vi "_testStepCfgEditor.vi"() -> ()   [LabVIEW 2010]
panel:
  out "View row details":string[](array[string])
  in  "stop":bool
  in  "Library function":string(tree)="sigDirMulStatInSet"
  in  "Test Step CFG EDIT":string[][](table)
  out "error out":errorcluster
  in  "error in":errorcluster
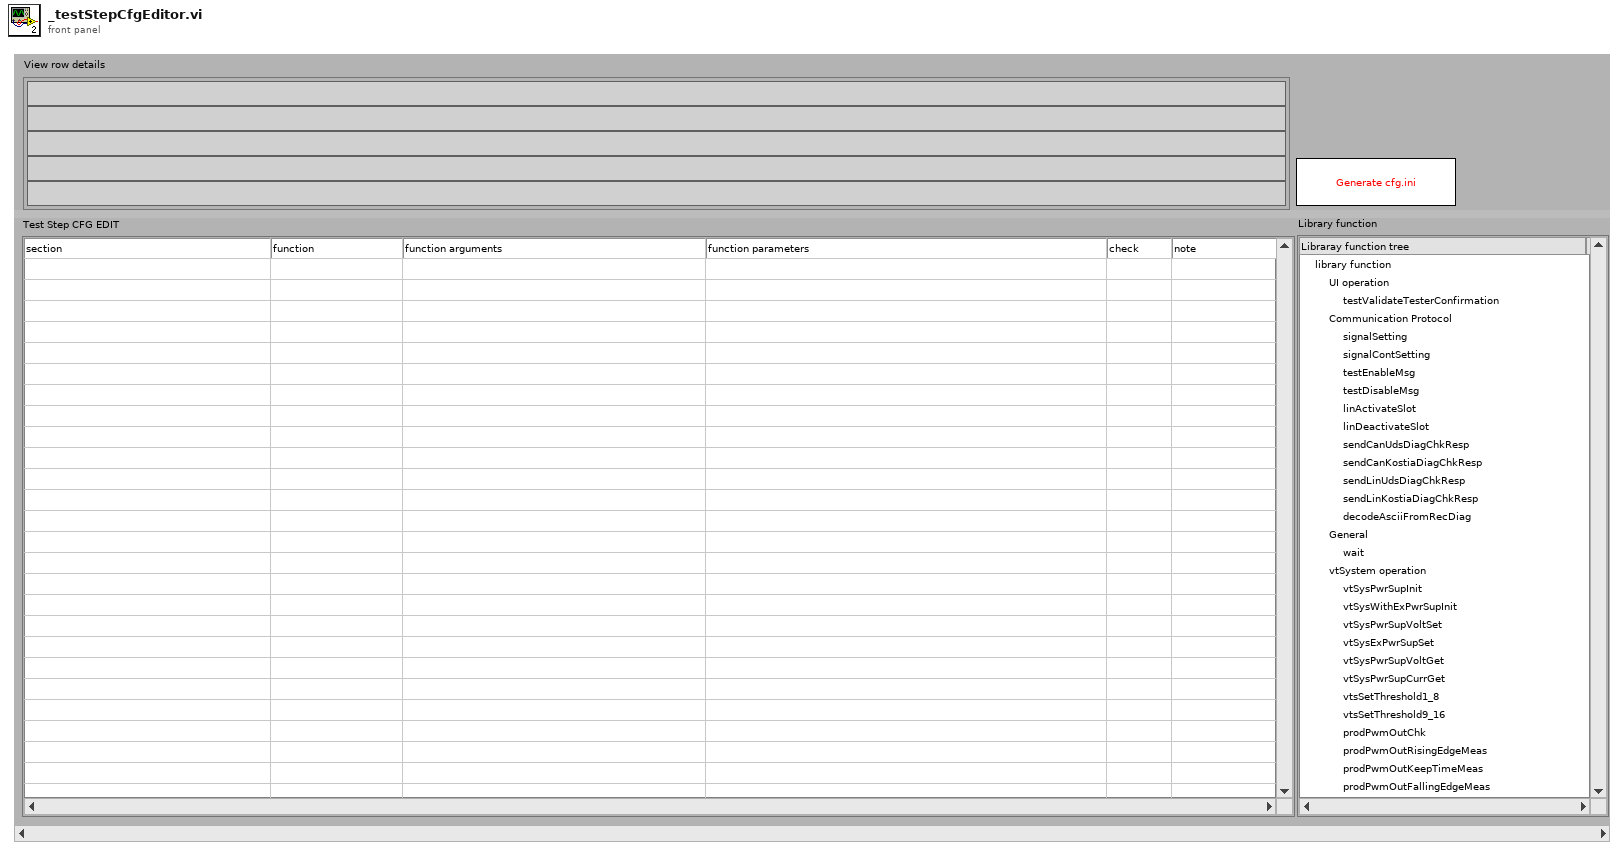
[diagram p1: front panel]
types:
  T1 = typedef "LVRowAndColumnTypeDef.ctl" = cluster{"Row":i32, "Column":i32}
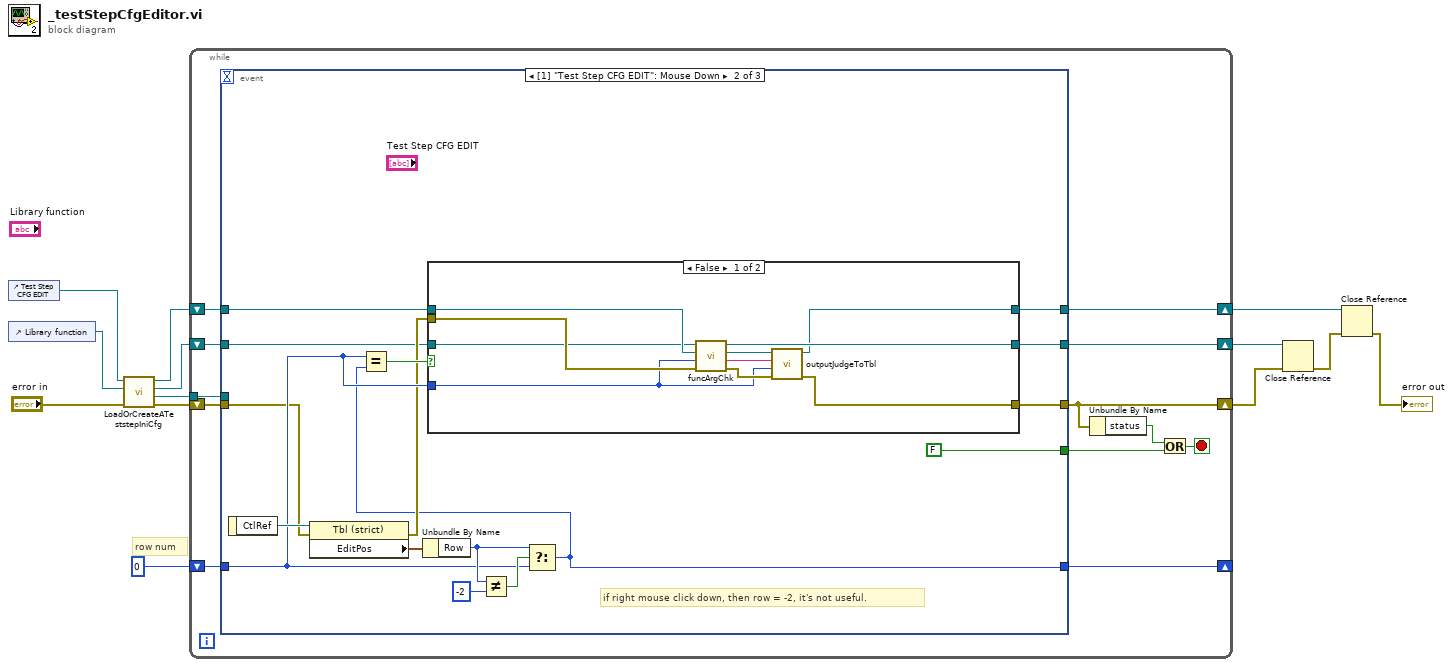
[diagram p0: block diagram]
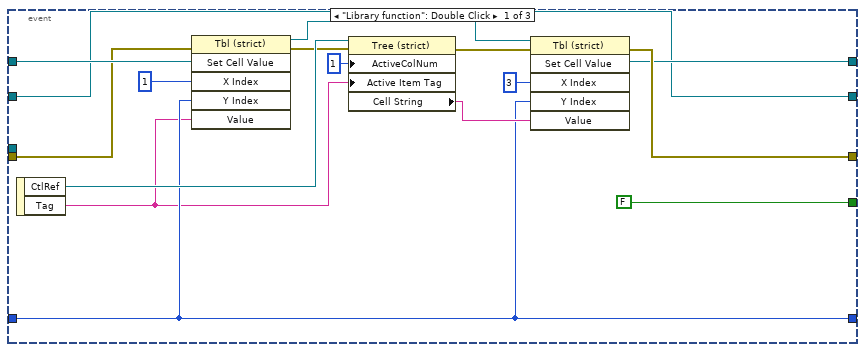
[diagram p2: hidden frame]
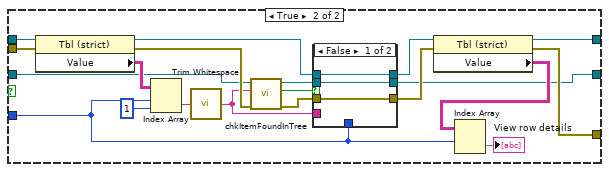
[diagram p3: hidden frame]
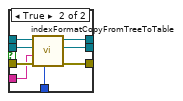
[diagram p4: hidden frame]
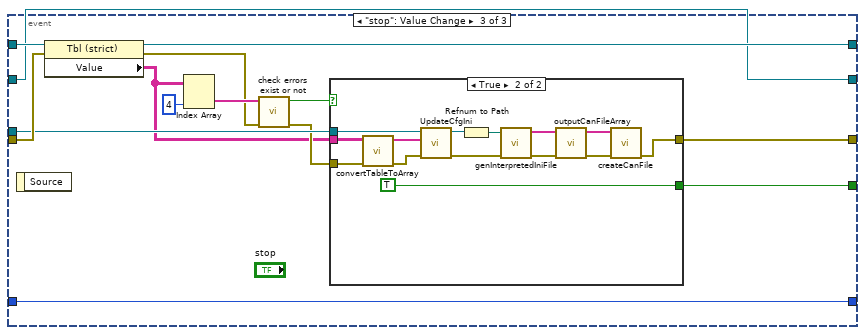
[diagram p5: hidden frame]
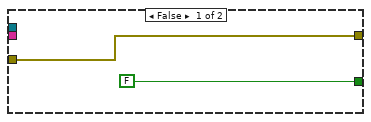
[diagram p6: hidden frame]
diagram:
  # "row num"
  n1 = control-ref of="Test Step CFG EDIT"() -> (w12:refnum<vi>)
  n2 = control-ref of="Library function"() -> (w13:refnum<vi>)
  n3 = call "LoadOrCreateATeststepIniCfg.vi"("error in"="error in", "Tree Refnum"=w13, "Tbl Refnum in"=w12) -> ("error out"=w6:errorcluster, "cfg file refnum out"=w10:refnum<file>, "Tree Refnum out"=w5:refnum<vi>, "Tbl Refnum out"=w7:refnum<vi>)  [unwired: 5 in]
  n4 = while {
    shift-right: [w22] -> w3
    shift-left: w6 -> [w25]
    shift-right: [w18] -> _
    shift-left: 0 ("Row") -> [w19]
    shift-right: [w17] -> w9
    shift-left: w7 -> [w20]
    tunnel: w10 -> [w16]
    shift-right: [w14] -> w4
    shift-left: w5 -> [w15]
    stop <- w23 stop-if-true
    n5 = event shown="[1] \"Test Step CFG EDIT\": Mouse Down" {
      selector: _ -> [_ _ _]
      dyn-events: _ -> [_ _ _]
      timeout: _ -> [_ _ _]
      tunnel: w25 -> [w40 w47 w108]
      tunnel: [w31 w52 w109] -> w22
      tunnel: [FALSE ("stop") FALSE ("stop") w112] -> w24
      tunnel: w20 -> [w41 w42 w110]
      tunnel: w19 -> [w29 w49 w111]
      tunnel: [w29 w43 w111] -> w18
      tunnel: [w28 w50 w103] -> w17
      tunnel: w16 -> [_ _ w107]
      tunnel: w15 -> [w27 w45 w99]
      tunnel: [w27 w44 w99] -> w14
      event "Library function": Double Click {
        n6 = event-data() -> ("CtlRef"=w38:refnum<vi>, "Tag"=w26:string)  [unwired: 1 in]
        n7 = invoke class="Tbl (strict)" method="Set Cell Value"(reference=w41, error in=w40, "X Index"=u32 1 ("Y Index"), "Y Index"=w29, "Value"=w26) -> (reference out=w32:refnum<vi>, error out=w33:errorcluster)  [unwired: 1 in, 4 out]
        n8 = property class="Tree (strict)"(reference=w38, error in=w33, "ActiveColNum"=1 ("Active Cell:Active Column Number"), "Active Item Tag"=w26) -> (error out=w36:errorcluster, "Cell String"=w35:string)  [unwired: 1 out]
        n9 = invoke class="Tbl (strict)" method="Set Cell Value"(reference=w32, error in=w36, "X Index"=u32 3, "Y Index"=w29, "Value"=w35) -> (reference out=w28:refnum<vi>, error out=w31:errorcluster)  [unwired: 1 in, 4 out]
      }
      event "Test Step CFG EDIT": Mouse Down {
        # "if right mouse click down, then row = -2, it's not useful."
        n10 = event-data() -> ("CtlRef"=w57:refnum<vi>)  [unwired: 1 in]
        n11 = property class="Tbl (strict)"(reference=w57, error in=w47) -> (error out=w46:errorcluster, "EditPos"=w56:T1)  [unwired: 1 out]
        n12 = Unbundle By Name(w56) -> ("Row"=w53:i32)
        n13 = Not Equal?(x=w53, y=-2) -> (x != y?=w54:bool)
        n14 = Select(t=w53, s=w54, f=w49) -> (s? t:f=w43:i32)
        n15 = Equal?(x=w49, y=w43) -> (x = y?=w51:bool)
        n16 = case shown="False" w51 {
          tunnel: w49 -> [w61 w71]
          tunnel: w42 -> [w66 w85]
          tunnel: w46 -> [w67 w84]
          tunnel: [w58 w77] -> w52
          tunnel: [w59 w86] -> w50
          tunnel: w45 -> [w65 w79]
          tunnel: [w64 w68] -> w44
          frame False {
            n17 = call "funcArgChk.vi"("error in"=w67, "Row number"=w61, "Tbl Refnum in"=w66, "Tree Refnum in"=w65) -> ("error out"=w62:errorcluster, "Check result"=w63:string, "Tbl Refnum out"=w60:refnum<vi>, "Tree Refnum out"=w64:refnum<vi>)  [unwired: 4 in]
            n18 = call "outputJudgeToTbl.vi"("error in"=w62, "rowNum"=w61, "judgeRes"=w63, "Tbl Refnum in"=w60) -> ("error out"=w58:errorcluster, "Tbl Refnum Out"=w59:refnum<vi>)  [unwired: 6 in]
          }
          frame True {
            n19 = property class="Tbl (strict)"(reference=w85, error in=w84) -> (reference out=w73:refnum<vi>, error out=w80:errorcluster, "Value"=w83:string[][])
            n20 = Index Array(array=w83, index (row)=w71, index (col)=1 ("disabled index (col)")) -> (element=w81:string)
            n21 = call <vilib>:"Trim Whitespace.vi"("string"=w81) -> ("trimmed string"=w72:string)  [unwired: 1 in]
            n22 = call "chkItemFoundInTree.vi"("error in"=w80, "searchItem"=w72, "Tree Refnum in"=w79) -> ("error out"=w76:errorcluster, "FoundInTree?"=w75:bool, "Tree Refnum out"=w74:refnum<vi>)  [unwired: 6 in]
            n23 = case shown="False" w75 {
              tunnel: [w90 w98] -> w70
              tunnel: [w88 w97] -> w69
              tunnel: w71 -> [_ w96]
              tunnel: [w89 w95] -> w68
              tunnel: w74 -> [w89 w94]
              tunnel: w76 -> [w88 w93]
              tunnel: w73 -> [w90 w92]
              tunnel: w72 -> [_ w91]
              frame False {
              }
              frame True {
                n24 = call "indexFormatCopyFromTreeToTable.vi"("rowNum"=w96, "error in"=w93, "searchItem"=w91, "Tree Refnum In"=w94, "Tbl Refnum in"=w92) -> ("error out"=w97:errorcluster, "Tree Refnum Out"=w95:refnum<vi>, "Tbl Refnum Out"=w98:refnum<vi>)  [unwired: 4 in]
              }
            }
            n25 = property class="Tbl (strict)"(reference=w70, error in=w69) -> (reference out=w86:refnum<vi>, error out=w77:errorcluster, "Value"=w78:string[][])
            n26 = Index Array(array=w78, index (row)=w71) -> (element=→"View row details":string[])  [unwired: 1 in]
          }
        }
      }
      event "stop": Value Change {
        n27 = event-data() -> ()  [unwired: 1 in, 1 out]
        n28 = property class="Tbl (strict)"(reference=w110, error in=w108) -> (reference out=w103:refnum<vi>, error out=w104:errorcluster, "Value"=w100:string[][])
        n29 = Index Array(array=w100, index (col)=4 ("disabled index (col)")) -> (element=w105:string[])  [unwired: 1 in]
        n30 = call "check errors exist or not.vi"("error in"=w104, "judge column"=w105) -> ("error out"=w102:errorcluster, "Go on?"=w101:bool)  [unwired: 8 in]
        n31 = case shown="True" w101 {
          tunnel: [FALSE ("stop") TRUE ("stop")] -> w112
          tunnel: [w113 w124] -> w109
          tunnel: w107 -> [_ w125]
          tunnel: w102 -> [w113 w127]
          tunnel: w100 -> [_ w121]
          frame False {
          }
          frame True {
            n32 = call "convertTableToArray.vi"("error in"=w127, "tbl"=w121) -> ("error out"=w126:errorcluster, "contArr"=w123:string[])  [unwired: 8 in]
            n33 = call "UpdateCfgIni.vi"("error in"=w126, "contentArray"=w123, "iniCfgRefnumIn"=w125) -> ("error out"=w119:errorcluster, "iniCfgRefnumOut"=w115:refnum<file>)  [unwired: 7 in]
            n34 = Refnum to Path(1:w115) -> (0:w116:path)
            n35 = call "genInterpretedIniFile.vi"("error in"=w119, "configuration file path"=w116) -> ("error out"=w118:errorcluster, "interpretedIniFileContentArray"=w117:string[])  [unwired: 8 in]
            n36 = call "outputCanFileArray.vi"("error in"=w118, "interpretedIniFileContentArray"=w117) -> ("error out"=w122:errorcluster, "testCaseInCanFileArr"=w120:string[])  [unwired: 8 in]
            n37 = call "createCanFile.vi"("error in"=w122, "contentArray"=w120) -> ("error out"=w124:errorcluster)  [unwired: 9 in]
          }
        }
      }
    }
    n38 = Unbundle By Name(w22) -> ("status"=w21:bool)
    n39 = Or(x=w21, y=w24) -> (x .or. y?=w23:bool)
  }
  n40 = Close Reference(reference=w4, error in (no error)=w3) -> (error out=w2:errorcluster)
  n41 = Close Reference(reference=w9, error in (no error)=w2) -> (error out=→"error out":errorcluster)
